vi "getSpecificTopic.vi"(8 "error in (no error)":errorcluster, 10 "nameTopic":string, 11 "Module in":refnum<class "Module.lvclass">) -> (0 "error out":errorcluster, 2 "Topic.lvclass":refnum<class "Topic.lvclass">, 3 "Module out":refnum<class "Module.lvclass">)   [LabVIEW 2018, in "Module.lvclass"]
doc: "Get the specific topic based on the topic's name."
uses:
  Module.lvclass
  Topic/Topic.lvclass
  Module.lvclass/Module.ctl
  Topic/Topic.lvclass/Topic.ctl
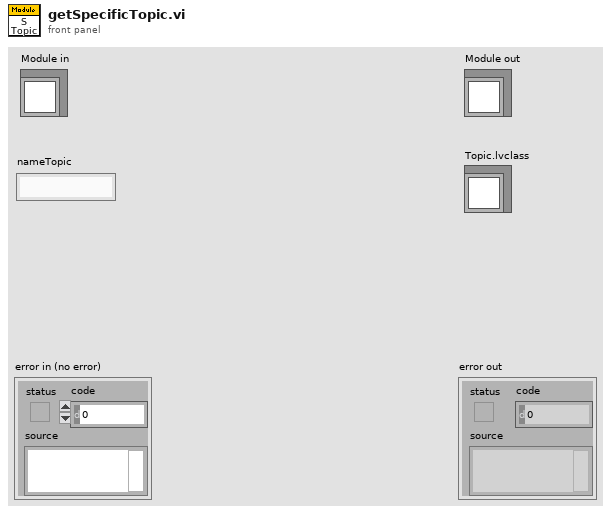
[diagram p1: front panel]
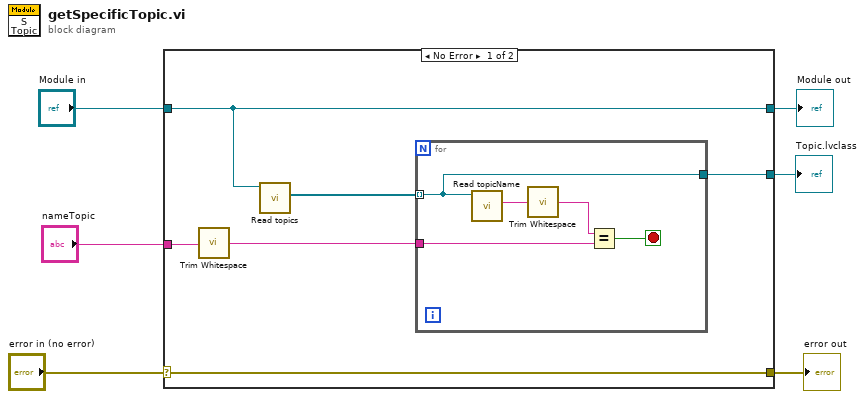
[diagram p0: block diagram]
diagram:
  n1 = case shown="No Error" "error in (no error)" {
    selector: "error in (no error)" -> [w12 w19]
    tunnel: [w12 w19] -> w5
    tunnel: [w9 w18] -> w3
    tunnel: "Module in" -> [w9 w18]
    tunnel: [w11 _] -> w2
    tunnel: "nameTopic" -> [w10 _]
    frame No Error {
      n2 = call <vilib>:"Trim Whitespace.vi"("string"=w10) -> ("trimmed string"=w7:string)  [unwired: 1 in]
      n3 = call "Read topics.vi"("Module in"=w9) -> ("topics"=w8:refnum<class "Topic.lvclass">[])  [unwired: 8 in, 2 out]
      n4 = for {
        tunnel: [w14] -> w11
        tunnel: w8 -> [w14] mode=indexing
        tunnel: w7 -> [w13]
        stop <- w16 stop-if-true
        n5 = call "Read topicName.vi"("Topic in"=w14) -> ("topicName"=w17:string)  [unwired: 8 in, 2 out]
        n6 = call <vilib>:"Trim Whitespace.vi"("string"=w17) -> ("trimmed string"=w15:string)  [unwired: 1 in]
        n7 = Equal?(x=w15, y=w13) -> (x = y?=w16:bool)
      }
    }
    frame Error {
    }
  }
  "error out" <- w5
  "Module out" <- w3
  "Topic.lvclass" <- w2
